vi "NonLinearController.vi"() -> ()   [LabVIEW 2019]
uses:
  <vilib>/NI/Modbus Library/API/Wrapper/Create Serial Master.vi
  <vilib>/NI/Modbus Library/API/Master/Modbus Master.lvclass
  <vilib>/addons/control/pid/pid.llb/PID (DBL).vi
  <vilib>/addons/control/pid/NI_PID_pid.lvlib
  <vilib>/NI/Modbus Library/API/Wrapper/API Main.lvlib
panel:
  out "Frecuencia":dbl(graph)
  in  "Ajuste":dbl=6.0
  out "VFD frecuencia\n(Hz)":dbl
  in  "Puerto VFD":refnum<visa-resource-name>="COM4"
  out "Velocidad\nmedida (rpm)":i32
  out "Voltaje \nmedido (Vrms)":dbl format="%#_4f"
  out "Corriente\nmedida (Irms)":dbl format="%#_4f"
  in  "PID constantes":T1={"proportional gain (Kc)"=0.675, "integral time (Ti, min)"=0.0, "derivative time (Td, min)"=0.0} {"derivative time (Td, min)" format="%.3f"; "integral time (Ti, min)" format="%.3f"; "proportional gain (Kc)" format="%.3f"}
  out "Velocidad rotorica":cluster{dbl, dbl}(graph)
  in  "Voltaje\ndeseado (Vrms)":dbl=125.0
  out "Velocidad \ndeseada (rpm)":dbl
  out "Voltaje":cluster{"Vd":dbl, dbl}(graph) caption="Waveform Chart"
  out "RL":dbl
  in  "Stop":bool
  # "Conexión\nde cargas"
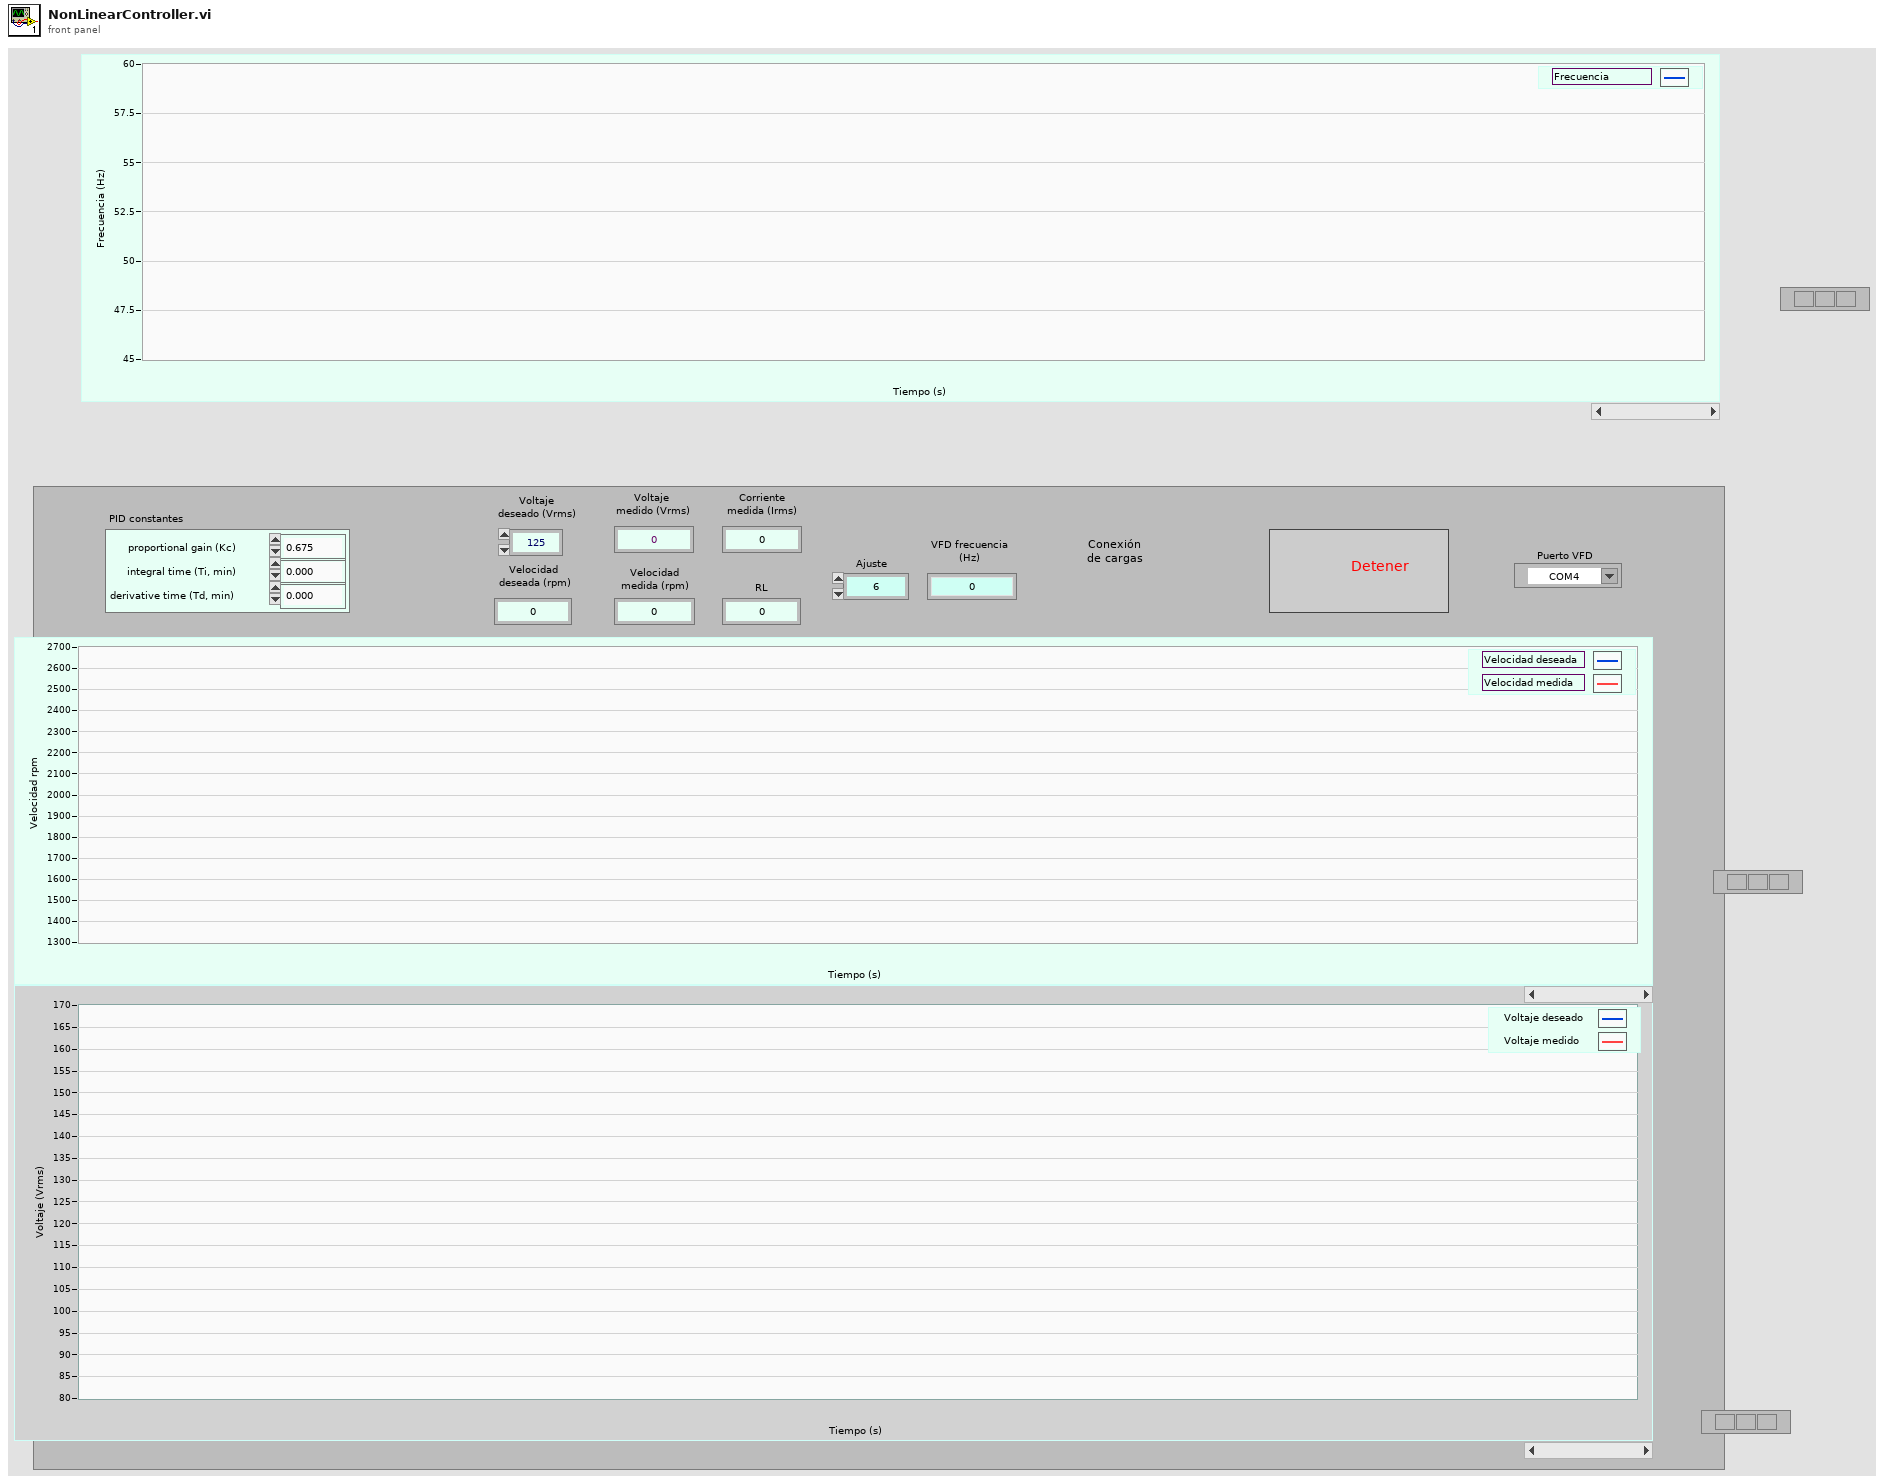
[diagram p1: front panel]
types:
  T1 = cluster{"proportional gain (Kc)":dbl, "integral time (Ti, min)":dbl, "derivative time (Td, min)":dbl}
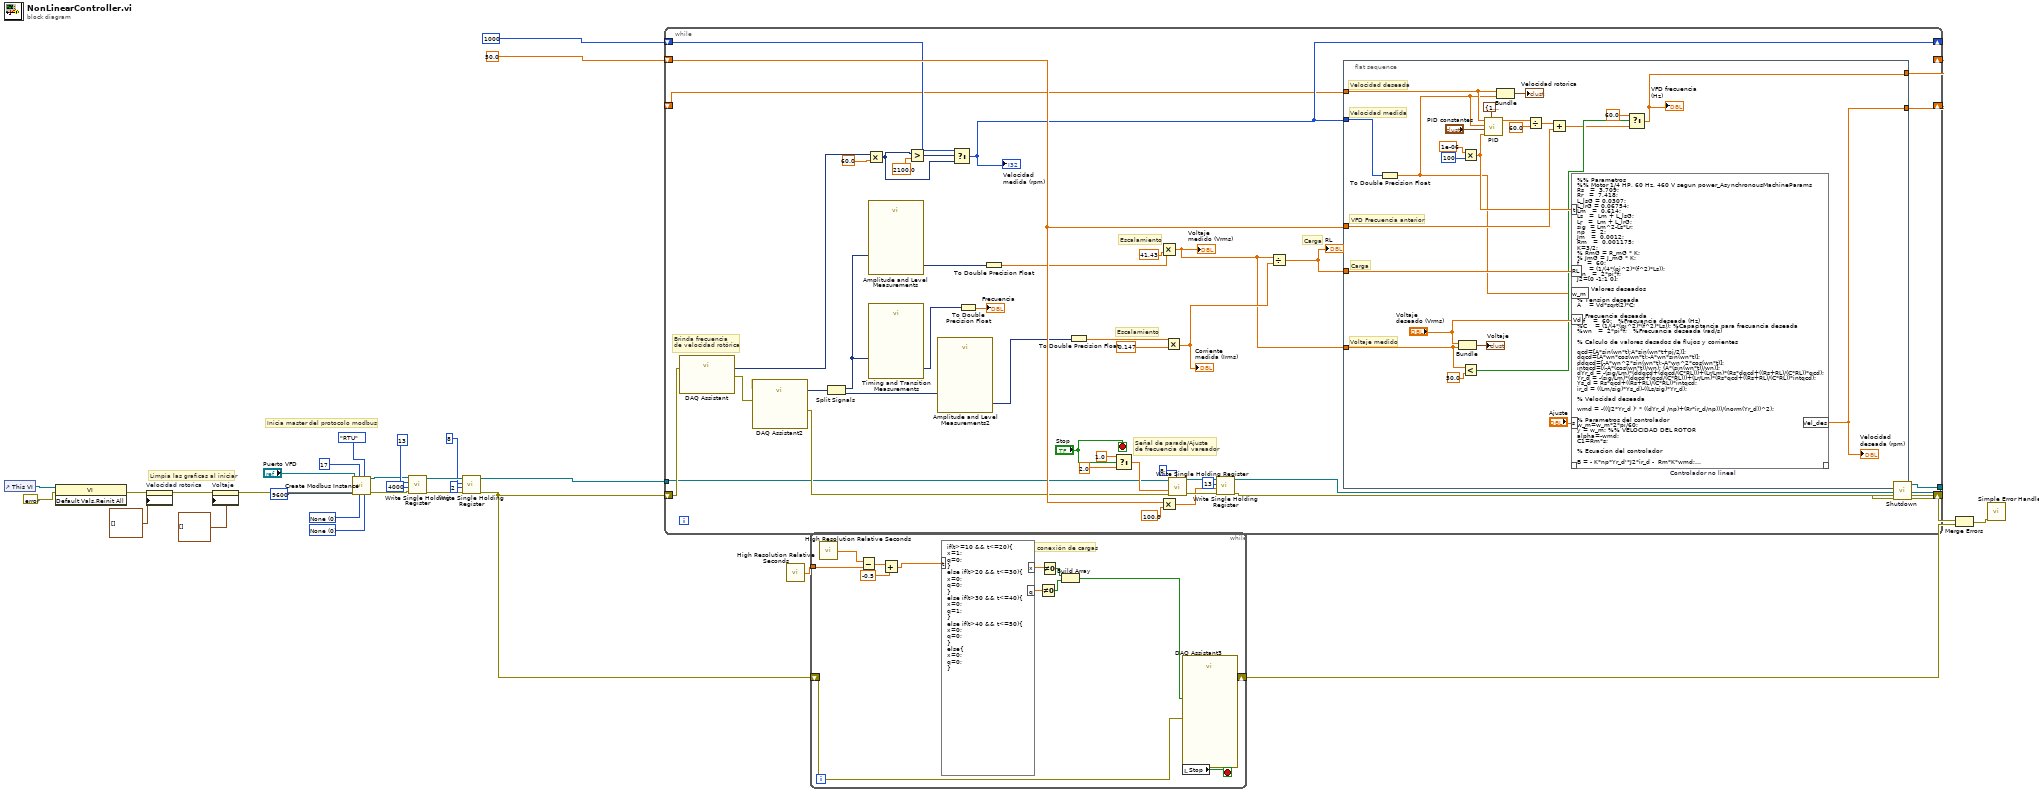
[diagram p0: block diagram]
diagram:
  w28 = u16 0 items=["None", "Odd", "Even", "Mark", "Space"] ("parity (even)")
  w29 = u16 0 items=["None", "XON/XOFF", "RTS/CTS", "XON/XOFF & RTS/CTS", "DTR/DSR", "XON/XOFF & DTR/DSR"] ("flow control (none)")
  # "Inicia master del protocolo modbus"
  # "Limpia las graficas al iniciar"
  n1 = control-ref of="This VI"() -> (w10:refnum<vi>)
  n2 = invoke class="VI" method="Default Vals.Reinit All"(reference=w10, error in=errorcluster {"status"=FALSE, "code"=0, "source"=""}) -> (error out=w8:errorcluster)  [unwired: 1 in, 2 out]
  n3 = property on="Velocidad rotorica" class="WFChart (strict)"(error in=w8, "History Data"=cluster{dbl, i32}[] []) -> (error out=w7:errorcluster)  [unwired: 1 in, 1 out]
  n4 = property on="Voltaje" class="WFChart (strict)"(error in=w7, "History Data"=cluster{"Vd":dbl, dbl}[] []) -> (error out=w6:errorcluster)  [unwired: 1 in, 1 out]
  n5 = call-poly <vilib>:"Create Modbus Instance.vi"("flow control (none)"=w29, "serial type"=enum16{"RTU", "ASCII"}."RTU", "parity (even)"=w28, "unit ID"=u8 17, "error in"=w6, "baud rate"=u32 9600, "VISA resource name"="Puerto VFD") -> ("error out"=w21:errorcluster, "serial master instance"=w22:refnum<class "Modbus Master.lvclass">)  [unwired: 3 in]
  n6 = call-dynamic "Write Single Holding Register.vi"("error in"=w21, "register to write"=u16 4000, "address"=u16 13 ("Frequency"), "Modbus master in"=w22) -> ("error out"=w13:errorcluster, "Modbus master out"=w14:refnum<class "Modbus Master.lvclass">)  [unwired: 6 in]
  n7 = call-dynamic "Write Single Holding Register.vi"("error in"=w13, "register to write"=u16 2, "address"=u16 8, "Modbus master in"=w14) -> ("error out"=w15:errorcluster, "Modbus master out"=w16:refnum<class "Modbus Master.lvclass">)  [unwired: 6 in]
  n8 = while {
    tunnel: w16 -> [w37]
    shift-right: [w61] -> _
    shift-left: 50.0 -> [w60]
    shift-right: [w55] -> _
    shift-left: 1000 -> [w56]
    shift-right: [w54] -> _
    shift-left: _ -> [w53]
    shift-right: [w36] -> w3
    shift-left: w15 -> [w46]
    tunnel: [w35] -> w2
    stop <- "Stop" stop-if-true
    # "Carga"
    # "Escalamiento"
    # "Escalamiento"
    # "Señal de parada/Ajuste \nde frecuencia del vareador"
    # "Lectura analógica"
    # "Brinda frecuencia\nde velocidad rotórica"
    n9 = call "DAQ Assistant"("error in"=w46) -> ("data"=w62:dynamicdata, "error out"=w45:errorcluster)  [unwired: 16 in, 1 out]
    n10 = call "DAQ Assistant2"("error in"=w45) -> ("data"=w64:dynamicdata, "error out"=w44:errorcluster)  [unwired: 15 in, 2 out]
    n11 = Split Signals(w64) -> (w34:dynamicdata, w40:dynamicdata)  [unwired: 2 in]
    n12 = Multiply(x=w62, y=60.0) -> (x*y=w57:dynamicdata)
    n13 = call "Amplitude and Level Measurements"("Signals"=w34) -> ("Positive Peak"=w42:dynamicdata)  [unwired: 13 in, 1 out]
    n14 = call "Timing and Transition Measurements"("Signals"=w34) -> ("Frequency"=w33:dynamicdata)  [unwired: 9 in, 1 out]
    n15 = Greater?(x=w57, y=2100.0) -> (0:w58:dynamicdata)
    n16 = call "Amplitude and Level Measurements2"("Signals"=w40) -> ("Positive Peak"=w39:dynamicdata)  [unwired: 13 in, 1 out]
    n17 = Select(t=w56, s=w58, f=w57) -> (s? t:f=w55:i32)
    "Velocidad\nmedida (rpm)" <- w55
    n18 = To Double Precision Float(number=w33) -> (double precision float=→"Frecuencia":dbl)
    n19 = To Double Precision Float(number=w42) -> (double precision float=w41:dbl)
    n20 = To Double Precision Float(number=w39) -> (double precision float=w38:dbl)
    n21 = Select(t=1.0, s="Stop", f=2.0) -> (s? t:f=w68:dbl)
    n22 = Multiply(x=w41, y=41.43) -> (x*y=w48:dbl)
    "Voltaje \nmedido (Vrms)" <- w48
    n23 = Multiply(x=w60, y=100.0) -> (x*y=w50:dbl)
    n24 = Multiply(x=w38, y=0.147) -> (x*y=w51:dbl)
    "Corriente\nmedida (Irms)" <- w51
    n25 = call-dynamic "Write Single Holding Register.vi"("error in"=w44, "register to write"=w68, "address"=u16 8 ("Start"), "Modbus master in"=w37) -> ("error out"=w69:errorcluster, "Modbus master out"=w70:refnum<class "Modbus Master.lvclass">)  [unwired: 6 in]
    n26 = call-dynamic "Write Single Holding Register.vi"("error in"=w69, "register to write"=w50, "address"=u16 13 ("Frequency"), "Modbus master in"=w70) -> ("error out"=w36:errorcluster, "Modbus master out"=w35:refnum<class "Modbus Master.lvclass">)  [unwired: 6 in]
    n27 = Divide(x=w48, y=w51) -> (x/y=w52:dbl)
    "RL" <- w52
    n28 = flat-sequence {
      tunnel: w55 -> [w86]
      tunnel: [w76] -> w61
      tunnel: w60 -> [w88]
      tunnel: w52 -> [w87]
      tunnel: [w73] -> w54
      tunnel: w53 -> [w84]
      tunnel: w48 -> [w81]
      frame #0 {
        # "VFD Frecuencia anterior"
        # "Velocidad medida"
        # "Carga"
        # "Voltaje medido"
        # "Velocidad deseada"
        n29 = To Double Precision Float(number=w86) -> (double precision float=w74:dbl)
        n30 = Bundle("Voltaje\ndeseado (Vrms)"="Voltaje\ndeseado (Vrms)", w81) -> (→"Voltaje":cluster{"Voltaje\ndeseado (Vrms)":dbl, dbl})  [unwired: 1 in]
        n31 = Multiply(x=1e-06, y=u32 100 ("millisecond multiple")) -> (x*y=w85:dbl)
        n32 = Less?(x=w81, y=50.0) -> (x < y?=w79:bool)
        n33 = call-poly <vilib>:"PID.vi"("output range"=cluster{"output high":dbl, "output low":dbl} {"output high"=100.0, "output low"=-100.0}, "dt (s)"=w85, "PID gains"="PID constantes", "process variable"=w74, "setpoint"=w84) -> ("output"=w91:dbl)  [unwired: 5 in, 1 out]
        n34 = Bundle(w84, w74) -> (→"Velocidad rotorica":cluster{dbl, dbl})  [unwired: 1 in]
        n35 = Divide(x=w91, y=60.0) -> (x/y=w89:dbl)
        n36 = Add(x=w89, y=w88) -> (x+y=w77:dbl)
        n37 = script code="%% Parametros\n%% Motor 1/4 HP, 60 Hz, 460 V segun power_AsynchronousMachineParams\nRs   =  3.709;\nRr   =  7.418;\nL_lsG = 0.0307;\nL_lrG = 0.06754;\nLm   =  0.614;\nLs   =  Lm + L_lsG;\nLr   =  Lm + L_lrG;\nsig  = Lm^2-Ls*Lr;\nnp   =  2;\nJm   =  0.0012;\nRm   =  0.001175; \nK=3/2;\n% RmG = R_mG * K;\n% JmG = J_mG * K;\nf    =  60;\nC    = (1/(4*(pi^2)*(f^2)*Ls));\nwn   =  2*pi*f;\nJ2=[0 -1;1 0];\n\n%% Valores deseados \n\n% Tension deseada \nA    = Vd*sqrt(2)*C;\n\n% Frecuencia deseada\n%f    =  60;\t\t\t%Frecuancia deseada (Hz)\n%C    = (1/(4*(pi^2)*(f^2)*Ls));\t%Capacitancia para frecuancia deseada\n%wn   =  2*pi*f;\t\t\t%Frecuancia deseada (rad/s)\n\n% Calculo de valores desados de flujos y corrientes\n\nqcd=[A*sin(wn*t);A*sin(wn*t+pi/2)];\ndqcd=[A*wn*cos(wn*t);-A*wn*sin(wn*t)];\nddqcd=[-A*wn^2*sin(wn*t);-A*wn^2*cos(wn*t)];\nintqcd=[(-A*(cos(wn*t))/wn); (A*(sin(wn*t))/wn)];\ndYr_d = -(sig/Lm)*(ddqcd+(dqcd/(C*RL)))+(Lr/Lm)*(Rs*dqcd+((Rs+RL)/(C*RL))*qcd);\nYr_d = -(sig/Lm)*(dqcd+(qcd/(C*RL)))+(Lr/Lm)*(Rs*qcd+((Rs+RL)/(C*RL))*intqcd);\nYs_d = Rs*qcd+((Rs+RL)/(C*RL))*intqcd;\nir_d = ((Lm/sig)*Ys_d)-((Ls/sig)*Yr_d);\n\n% Velocidad deseada\n\nwmd = -(((J2*Yr_d )' * ((dYr_d /np)+(Rr*ir_d/np)))/(norm(Yr_d))^2);\n\n% Parametros del controlador\nw_m=w_m*2*pi/60;\ny = w_m; %% VELOCIDAD DEL ROTOR\nalpha=-wmd;\nC1=Rm*s;\n\n% Ecuacion del controlador\n\nB = - K*np*Yr_d'*J2*ir_d -  Rm*K*wmd;\n\n% Controlador \nu = -B - C1*(y+alpha);\n\n\nVel_des= 60*u^2+212.8*u+1371.5;  \n%%Vel_des= 311.5*u+1334" "Controlador no lineal"("Vd"="Voltaje\ndeseado (Vrms)", "RL"=w87, "w_m"=w74, "t"=w85, "s"="Ajuste") -> ("Vel_des"=w73:dbl)  [unwired: 1 in, 1 out]
        "Velocidad \ndeseada (rpm)" <- w73
        n38 = Select(t=60.0, s=w79, f=w77) -> (s? t:f=w76:dbl)
        "VFD frecuencia\n(Hz)" <- w76
      }
    }
  }
  n39 = call <vilib>:"High Resolution Relative Seconds.vi"() -> ("relative seconds"=w1:dbl)
  n40 = while {
    shift-right: [w109] -> w19
    shift-left: w15 -> [w108]
    tunnel: w1 -> [w100]
    stop <- w107 stop-if-true
    # "Bloque para conexión de cargas"
    n41 = call <vilib>:"High Resolution Relative Seconds.vi"() -> ("relative seconds"=w101:dbl)
    n42 = Subtract(x=w101, y=w100) -> (x-y=w99:dbl)
    n43 = Add(x=w99, y=-0.5) -> (x+y=w97:dbl)
    n44 = formula code="if(t>=10 && t<=20){\nx=1;\nq=0;\n}\nelse if(t>20 && t<=30){\nx=0;\nq=0;\n}\nelse if(t>30 && t<=40){\nx=0;\nq=1;\n}\nelse if(t>40 && t<=50){\nx=0;\nq=0;\n}\nelse{\nx=0;\nq=0;\n}"("t"=w97) -> ("x"=w106:dbl, "q"=w105:dbl)
    n45 = Not Equal To 0?(x=w105) -> (x != 0?=w103:bool)
    n46 = Not Equal To 0?(x=w106) -> (x != 0?=w104:bool)
    n47 = Build Array(w104, w103) -> (w102:bool[])
    n48 = call "DAQ Assistant3"("data"=w102, "error in"=w108) -> ("error out"=w109:errorcluster)  [unwired: 16 in, 1 out]
    n49 = local read "Stop"() -> (w107:bool)
  }
  n50 = call-dynamic "Shutdown.vi"("error in"=w3, "Modbus master in"=w2) -> ("error out"=w18:errorcluster)  [unwired: 9 in]
  n51 = Merge Errors(w18, w19) -> (w17:errorcluster)
  n52 = call <vilib>:"Simple Error Handler.vi"("error in (no error)"=w17) -> ()  [unwired: 4 in, 5 out]
